vi "Encoders.vi"(0 "Reset Encoders?":bool) -> (3 "Total Distance":dbl, 4 "Avg Rate":dbl, 5 "X Distance":dbl, 6 "Y Distance":dbl)   [LabVIEW 2016, in "Apple script.lvlib"]
uses:
  Apple script.lvlib
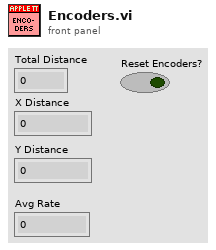
[diagram p1: front panel]
types:
  T1 = typedef "WPI_EncoderDevRef.ctl" = cluster{"DevStatus":errorcluster, "EncoderIndex":T2, "CounterIndex":T3, "DistancePerCount":dbl, "Decoding Type":T4}
  T2 = typedef "FPGA_EncoderIdx.ctl" = enum8{"Enc 0", "Enc 1", "Enc 2", "Enc 3", "Enc 4", "Enc 5", "Enc 6", "Enc 7", "Invalid"}
  T3 = typedef "FPGA_CounterCtrSystemIndex.ctl" = enum8{"Ctr 0", "Ctr 1", "Ctr 2", "Ctr 3", "Ctr 4", "Ctr 5", "Ctr 6", "Ctr 7", "Invalid"}
  T4 = typedef "WPI_EncoderType.ctl" = enum16{"1x", "2x", "4x"}
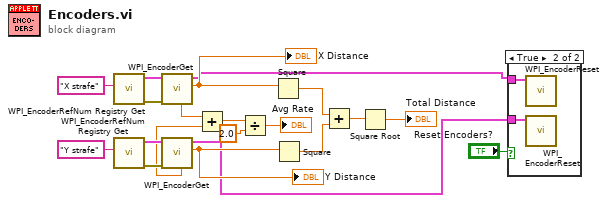
[diagram p0: block diagram]
diagram:
  n1 = call <vilib>:"WPI_EncoderRefNum Registry Get.vi"("refnum name"="X strafe") -> ("error out"=w20:errorcluster, "EncoderDevRef"=w19:T1)  [unwired: 9 in]
  n2 = call <vilib>:"WPI_EncoderRefNum Registry Get.vi"("refnum name"="Y strafe") -> ("error out"=w15:errorcluster, "EncoderDevRef"=w16:T1)  [unwired: 9 in]
  n3 = call <vilib>:"WPI_EncoderGet.vi"("error in (no error)"=w20, "EncoderDevRef"=w19) -> ("Distance"=w10:dbl, "EncoderDevRef"=w2:T1, "Rate"=w7:dbl)  [unwired: 4 in, 3 out]
  "X Distance" <- w10
  n4 = call <vilib>:"WPI_EncoderGet.vi"("error in (no error)"=w15, "EncoderDevRef"=w16) -> ("Distance"=w14:dbl, "EncoderDevRef"=w3:T1, "Rate"=w6:dbl)  [unwired: 4 in, 3 out]
  "Y Distance" <- w14
  n5 = Add(x=w7, y=w6) -> (x+y=w8:dbl)
  n6 = Divide(x=w8, y=2.0) -> (x/y=→"Avg Rate":dbl)
  n7 = Square(x=w10) -> (x^2=w12:dbl)
  n8 = Square(x=w14) -> (x^2=w11:dbl)
  n9 = Add(x=w12, y=w11) -> (x+y=w13:dbl)
  n10 = Square Root(x=w13) -> (sqrt(x)=→"Total Distance":dbl)
  n11 = case shown="True" "Reset Encoders?" {
    tunnel: w3 -> [_ w22]
    tunnel: w2 -> [_ w21]
    frame False {
    }
    frame True {
      n12 = call <vilib>:"WPI_EncoderReset.vi"("EncoderDevRef"=w21) -> ()  [unwired: 9 in, 2 out]
      n13 = call <vilib>:"WPI_EncoderReset.vi"("EncoderDevRef"=w22) -> ()  [unwired: 9 in, 2 out]
    }
  }
